vi "Error output.vi"(1 "I32 err code":i32) -> (0 "Error Out":errorcluster)   [LabVIEW 2014]
panel:
  # "PN 04/11/2014"
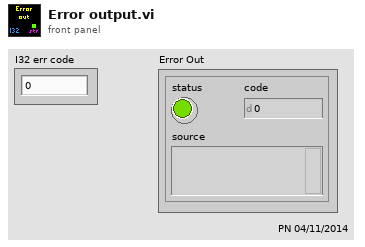
[diagram p1: front panel]
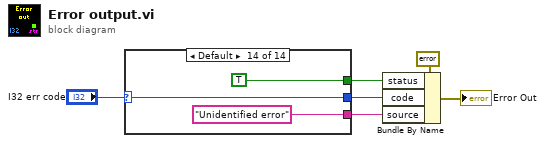
[diagram p0: block diagram]
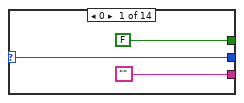
[diagram p2: hidden frame]
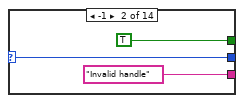
[diagram p3: hidden frame]
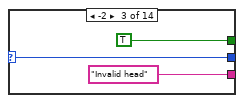
[diagram p4: hidden frame]
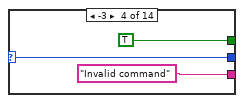
[diagram p5: hidden frame]
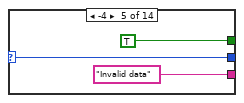
[diagram p6: hidden frame]
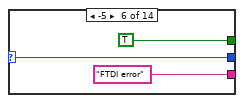
[diagram p7: hidden frame]
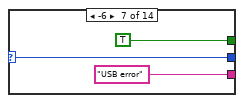
[diagram p8: hidden frame]
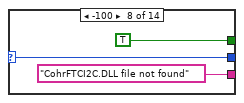
[diagram p9: hidden frame]
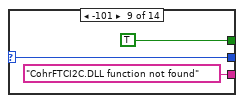
[diagram p10: hidden frame]
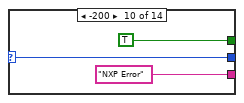
[diagram p11: hidden frame]
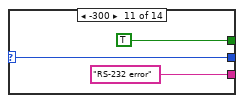
[diagram p12: hidden frame]
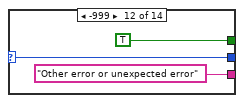
[diagram p13: hidden frame]
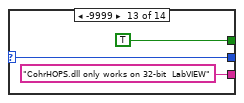
[diagram p14: hidden frame]
diagram:
  n1 = case shown="Default" "I32 err code" {
    selector: "I32 err code" -> [w8 w10 w13 w17 w19 w22 w25 w28 w31 w34 w37 w40 w43 w47]
    tunnel: ["" "Invalid handle" "Invalid head" "Invalid command" "Invalid data" "FTDI error" "USB error" "CohrFTCI2C.DLL file not found" "CohrFTCI2C.DLL function not found" "NXP Error" "RS-232 error" "Other error or unexpected error" "CohrHOPS.dll only works on 32-bit  LabVIEW" "Unidentified error"] -> w2
    tunnel: [w8 w10 w13 w17 w19 w22 w25 w28 w31 w34 w37 w40 w43 w47] -> w3
    tunnel: [FALSE TRUE TRUE TRUE TRUE TRUE TRUE TRUE TRUE TRUE TRUE TRUE TRUE TRUE] -> w1
    frame 0 {
    }
    frame -1 {
    }
    frame -2 {
    }
    frame -3 {
    }
    frame -4 {
    }
    frame -5 {
    }
    frame -6 {
    }
    frame -100 {
    }
    frame -101 {
    }
    frame -200 {
    }
    frame -300 {
    }
    frame -999 {
    }
    frame -9999 {
    }
    frame Default {
    }
  }
  n2 = Bundle By Name(cluster=errorcluster {"status"=FALSE, "code"=0, "source"=""} ("error constant"), "status"=w1, "code"=w3, "source"=w2) -> (→"Error Out":errorcluster)
